vi "create rxtx.vi"(8 "error in (no error)":errorcluster, 9 "qeue name":string, 10 "remote IP":string, 11 "Server in":refnum<class "Server.lvclass">) -> (0 "error out":errorcluster, 3 "Server out":refnum<class "Server.lvclass">)   [LabVIEW 2018, in "Server.lvclass"]
uses:
  Server.lvclass
  Server.lvclass/Server.ctl
  RxTx/RxTx.lvclass
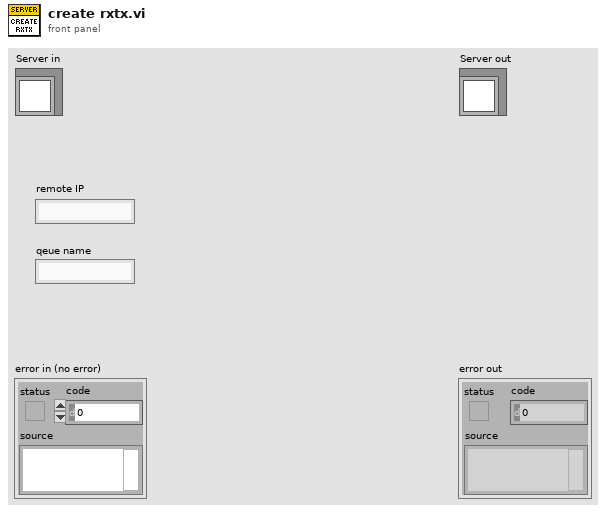
[diagram p1: front panel]
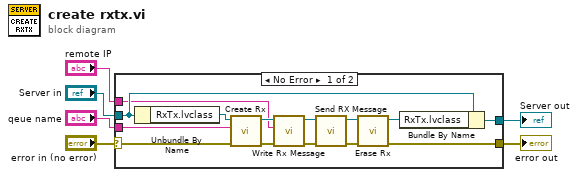
[diagram p0: block diagram]
diagram:
  n1 = case shown="No Error" "error in (no error)" {
    selector: "error in (no error)" -> [w10 w22]
    tunnel: [w9 w22] -> w5
    tunnel: [w11 w21] -> w3
    tunnel: "Server in" -> [w13 w21]
    tunnel: "remote IP" -> [w8 _]
    tunnel: "qeue name" -> [w7 _]
    frame No Error {
      n2 = Unbundle By Name(w13) -> ("RxTx.lvclass"=w14:refnum<class "RxTx.lvclass">)
      n3 = call "Create Rx.vi"("error in (no error)"=w10, "Reader Name"=w7, "RxTx in"=w14) -> ("error out"=w20:errorcluster, "RxTx out"=w17:refnum<class "RxTx.lvclass">)  [unwired: 7 in]
      n4 = call "Write Rx Message.vi"("error in (no error)"=w20, "Rx Message"=w8, "RxTx in"=w17) -> ("error out"=w19:errorcluster, "RxTx out"=w18:refnum<class "RxTx.lvclass">)  [unwired: 7 in]
      n5 = call "Send RX Message.vi"("error in (no error)"=w19, "RxTx in"=w18) -> ("error out"=w16:errorcluster, "RxTx out"=w15:refnum<class "RxTx.lvclass">)  [unwired: 8 in]
      n6 = call "Erase Rx.vi"("error in (no error)"=w16, "RxTx in"=w15) -> ("error out"=w9:errorcluster, "RxTx out"=w12:refnum<class "RxTx.lvclass">)  [unwired: 8 in]
      n7 = Bundle By Name(cluster=w13, "RxTx.lvclass"=w12) -> (w11:refnum<class "Server.lvclass">)
    }
    frame Error {
    }
  }
  "error out" <- w5
  "Server out" <- w3
